vi "ChangeGrating.vi"(8 "error in (no error)":errorcluster, 10 "Grating":enum16{"Mirror", "1200 g/mm", "1800 g/mm"}(ring), 11 "DongWoo in":refnum<class "DongWoo.lvclass">) -> (0 "error out":errorcluster, 3 "DongWoo out":refnum<class "DongWoo.lvclass">)   [LabVIEW 2023, in "DongWoo_Spectrometer.lvlib" / "DongWoo.lvclass"]
uses:
  DongWoo.lvclass
  DongWoo.lvclass/DongWoo.ctl
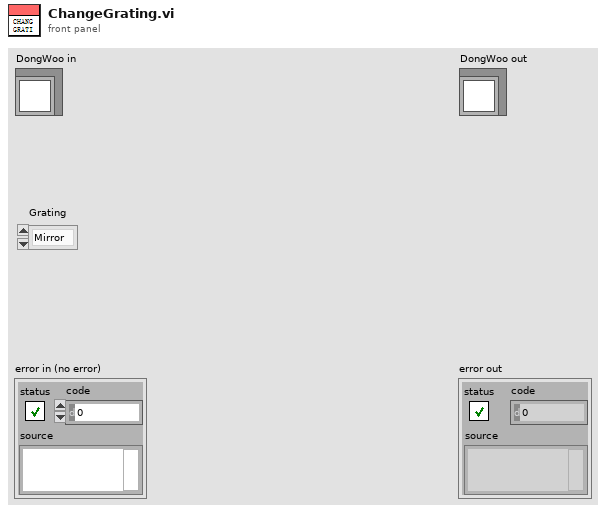
[diagram p1: front panel]
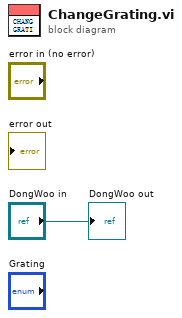
[diagram p0: block diagram]
diagram:
  "DongWoo out" <- "DongWoo in"
